vi "Uninit.vi"(11 "Test Caller Actor in":refnum<class "Test Caller Actor.lvclass">) -> (3 "Test Caller Actor out":refnum<class "Test Caller Actor.lvclass">)   [LabVIEW 2023, in "Test Caller Actor.lvlib" / "Test Caller Actor.lvclass"]
doc: "This method is the inverse of the Pre Launch Init.vi. This method is called unconditionally at the end of an actor's lifetime, even if there was an error in Pre Launch Init.vi. Note that the self Enqueuer for the actor is already invalid by the time this VI executes: within this method, the actor may send messages to its caller but not to itself. This method executes before Last Ack is sent.\n\nThis method neither receives nor produces an error cluster. It is designed to provide an unconditional release of acquired resources. Any error raised during release is considered to be irrelevant to the actor's lifetime. If the actor truly needs to report some error status, it may send a message to caller or include information within itself that callers can examine when handling Last Ack."
uses:
  Test Caller Actor.lvclass
  Test Caller Actor.lvclass/Test Caller Actor.ctl
  <userlib>/_OpenG.lib/error/error.llb/openg_error.lvlib
  <vilib>/ActorFramework/Actor/Actor.lvclass
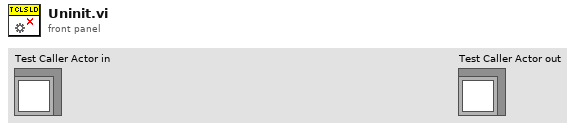
[diagram p1: front panel]
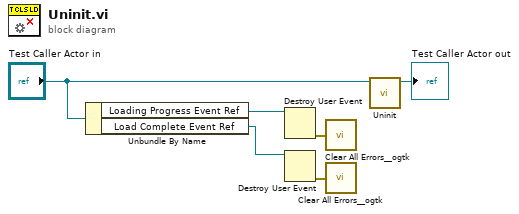
[diagram p0: block diagram]
diagram:
  n1 = Unbundle By Name("Test Caller Actor in") -> ("Loading Progress Event Ref"=w4:refnum<user-event>, "Load Complete Event Ref"=w1:refnum<user-event>)
  n2 = Destroy User Event(user event=w4) -> (error out=w3:errorcluster)  [unwired: 1 in]
  n3 = Destroy User Event(user event=w1) -> (error out=w2:errorcluster)  [unwired: 1 in]
  n4 = call <userlib>:"Clear All Errors__ogtk.vi"("Error In"=w3) -> ()  [unwired: 3 in, 1 out]
  n5 = call <userlib>:"Clear All Errors__ogtk.vi"("Error In"=w2) -> ()  [unwired: 3 in, 1 out]
  n6 = call-parent "Uninit.vi"("Actor in"="Test Caller Actor in") -> ("Actor out"=→"Test Caller Actor out":refnum<class "Test Caller Actor.lvclass">)  [unwired: 10 in]
